vi "basic array manipulation.vi"() -> ()   [LabVIEW 2016]
panel:
  out "z 2":dbl[][](array[numeric])
  out "z 1":dbl[][](array[numeric])
  in  "y":dbl[][](array[numeric])
  in  "x":dbl[][](array[numeric])
  out "c":dbl[](array[numeric])
  in  "b":dbl[](array[numeric])
  in  "a":dbl[](array[numeric])
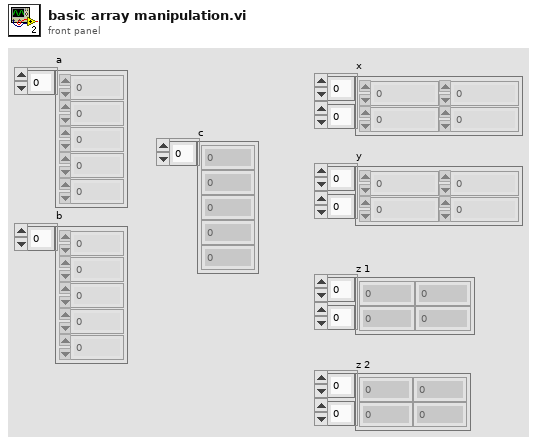
[diagram p1: front panel]
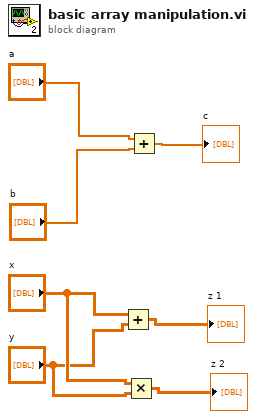
[diagram p0: block diagram]
diagram:
  n1 = Add(x="x", y="y") -> (x+y=→"z 1":dbl[][])
  n2 = Multiply(x="x", y="y") -> (x*y=→"z 2":dbl[][])
  n3 = Add(x="a", y="b") -> (x+y=→"c":dbl[])
